vi "AppendHeadersToArray.vi"(11 "Array":string[][](array[string])) -> (3 "output array":string[][](array[string]))   [LabVIEW 2013]
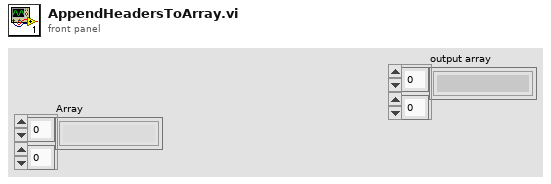
[diagram p1: front panel]
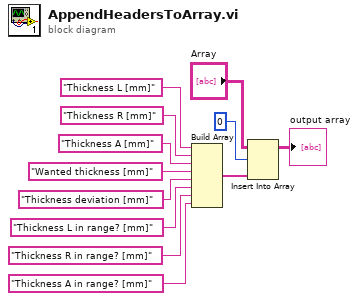
[diagram p0: block diagram]
diagram:
  n1 = Build Array("Thickness L [mm]", "Thickness R [mm]", "Thickness A [mm]", "Wanted thickness [mm]", "Thickness deviation [mm]", "Thickness L in range? [mm]", "Thickness R in range? [mm]", "Thickness A in range? [mm]") -> (w6:string[])
  n2 = Insert Into Array(array="Array", index (row)=0, new element=w6) -> (→"output array":string[][])  [unwired: 1 in]
